vi "CalcStepUncertainty.vi"(8 "error in (no error)":errorcluster, 10 "Limits":dbl[][][](array[numeric])=[[[0.059450168900494, 0.0606065605190911, 0.056793034460449, 0.0377791964132806, 0.0387680244678906, 0.041509529284321, 0.0, 0.0], [0.0543254248656728, 0.0605582232708396, 0.0705532258276927, 0.0403341376210629, 0.0362750710120636, 0.037641124860868, 0.0, 0.0], [0.0542535208152999, 0.0601149006696316, 0.057100190511556, 0.0286705153398605, 0.0306659503421681, 0.0318434771124804, 0.0, 0.0], [0.0539806772823237, 0.060111916581221, 0.0568149701475802, 0.0287477348403936, 0.030687681069202, 0.0318140233011936, 0.0, 0.0], [0.0574739206185427, 0.0628177175852463, 0.0608742935192014, 0.0507031710323209, 0.0492196025001063, 0.0512494967622953, 0.0, 0.0], [0.0573743399751993, 0.0636926206100454, 0.0626583117825458, 0.0369031527657219, 0.0385466857090226, 0.0400368175447213, 0.0, 0.0], [0.0831820808794742, 0.0842623844587226, 0.088262229564689, 0.0667743079383481, 0.0680308099651913, 0.0679787518894359, 0.0, 0.0], [0.0541037185786453, 0.0597178605956032, 0.0641248041876747, 0.0281653525639868, 0.0301909812864416, 0.0304719216326717, 0.0, 0.0], [0.0564462783136314, 0.0600214622402702, 0.0759912985981658, 0.0281162118220652, 0.0301892901163339, 0.0303638978137465, 0.0, 0.0], [0.0540653703792215, 0.0598738420777627, 0.0612858805251609, 0.0282196395706911, 0.0301950277548319, 0.0310242020330342, 0.0, 0.0], [0.056709051486753, 0.0602058925674664, 0.0806981932623049, 0.0281451428430134, 0.0302542048015808, 0.0304691904137436, 0.0, 0.0]]], 11 "Uncertainties":dbl[][][](array[numeric])=[[[0.059450168900494, 0.0606065605190911, 0.056793034460449, 0.0377791964132806, 0.0387680244678906, 0.041509529284321, 0.0, 0.0], [0.0543254248656728, 0.0605582232708396, 0.0705532258276927, 0.0403341376210629, 0.0362750710120636, 0.037641124860868, 0.0, 0.0], [0.0542535208152999, 0.0601149006696316, 0.057100190511556, 0.0286705153398605, 0.0306659503421681, 0.0318434771124804, 0.0, 0.0], [0.0539806772823237, 0.060111916581221, 0.0568149701475802, 0.0287477348403936, 0.030687681069202, 0.0318140233011936, 0.0, 0.0], [0.0574739206185427, 0.0628177175852463, 0.0608742935192014, 0.0507031710323209, 0.0492196025001063, 0.0512494967622953, 0.0, 0.0], [0.0573743399751993, 0.0636926206100454, 0.0626583117825458, 0.0369031527657219, 0.0385466857090226, 0.0400368175447213, 0.0, 0.0], [0.0831820808794742, 0.0842623844587226, 0.088262229564689, 0.0667743079383481, 0.0680308099651913, 0.0679787518894359, 0.0, 0.0], [0.0541037185786453, 0.0597178605956032, 0.0641248041876747, 0.0281653525639868, 0.0301909812864416, 0.0304719216326717, 0.0, 0.0], [0.0564462783136314, 0.0600214622402702, 0.0759912985981658, 0.0281162118220652, 0.0301892901163339, 0.0303638978137465, 0.0, 0.0], [0.0540653703792215, 0.0598738420777627, 0.0612858805251609, 0.0282196395706911, 0.0301950277548319, 0.0310242020330342, 0.0, 0.0], [0.056709051486753, 0.0602058925674664, 0.0806981932623049, 0.0281451428430134, 0.0302542048015808, 0.0304691904137436, 0.0, 0.0]]]) -> (0 "error out":errorcluster, 1 "clDlyTime":T1, 2 "clOvrUndr":T2={"OvrUndr"=[[[[[5.598492295160192, 5.589160017980474, 5.579827740800756, 6.2090278478135055, 6.202935187769419, 6.196842527725332, 6.270368754436869, 6.261733208094874, 6.2530976617528795, 5.499241138114173, 5.4912209769255735, 5.483200815736974, 5.591363005137677, 5.589161707344972, 5.586960409552266, 6.2034021327898525, 6.2029551231392706, 6.202508113488689, 6.262186470202315, 6.261747037530138, 6.261307604857961, 5.492149609028501, 5.491120362323346, 5.490091115618191], [4.582281382800085, 4.572949105620367, 4.563616828440649, 2.0737377226338936, 2.0676450625898064, 2.0615524025457193, 1.1136472889469742, 1.1050117426049793, 1.0963761962629843, 4.500837324127726, 4.492817162939127, 4.484797001750527, 4.57515178562041, 4.572950487827704, 4.570749190034999, 2.068098717363672, 2.06765170771309, 2.067204698062508, 1.1054536157657309, 1.1050141830935536, 1.1045747504213763, 4.493764088606066, 4.492734841900911, 4.491705595195756], [6.26023399342542, 6.250901716245702, 6.241569439065984, 6.128438171518977, 6.12234551147489, 6.116252851430803, 6.430675694174775, 6.422040147832781, 6.413404601490786, 6.102855597590311, 6.094835436401712, 6.086815275213112, 6.253149166340811, 6.2509478685481055, 6.2487465707554, 6.122858708702316, 6.122411699051734, 6.121964689401152, 6.422526817417168, 6.422087384744991, 6.421647952072814, 6.095816462969536, 6.094787216264381, 6.093757969559226], [3.375202432081235, 3.3658701549015175, 3.3565378777218, 3.302740243145951, 3.296647583101864, 3.2905549230577766, 1.1419367489007164, 1.1333012025587215, 1.1246656562167265, 2.0396319733224955, 2.0316118121338955, 2.0235916509452956, 3.368096303933992, 3.3658950061412862, 3.3636937083485803, 3.297130232216894, 3.296683222566312, 3.29623621291573, 1.1337489711565862, 1.133309538484409, 1.1328701058122317, 2.0326249854599556, 2.0315957387548007, 2.030566492049646]], [[5.6114389386325305, 5.602495822485004, 5.593552706337477, 6.4971644746473425, 6.4906779148884395, 6.4841913551295365, 6.452789687138199, 6.442635198982573, 6.432480710826947, 5.499700075652654, 5.491172020965302, 5.4826439662779505, 5.604365790119637, 5.602470106718821, 5.600574423318005, 6.491501742716185, 6.490751963178685, 6.4900021836411845, 6.443115798655941, 6.442548550239463, 6.4419813018229855, 5.492187667629821, 5.4911167638448894, 5.490045860059958], [4.592803334544344, 4.583860218396818, 4.574917102249291, 1.1519003094451032, 1.1454137496861998, 1.1389271899272964, 2.1576995544831505, 2.147545066327524, 2.1373905781718974, 4.501305162749851, 4.4927771080625, 4.484249053375148, 4.585734861625306, 4.58383917822449, 4.5819434948236735, 1.146176596569033, 1.1454268170315325, 1.144677037494032, 2.148083431829625, 2.1475161834131473, 2.1469489349966695, 4.4938028014762015, 4.49273189769127, 4.491660993906338], [5.824200079831354, 5.815256963683828, 5.806313847536301, 6.213851725577966, 6.207365165819063, 6.20087860606016, 6.175131282852548, 6.164976794696922, 6.154822306541296, 6.103387438698514, 6.094859384011162, 6.08633132932381, 5.81714404673894, 5.815248363338124, 5.813352679937307, 6.208174990295637, 6.207425210758137, 6.206675431220637, 6.165428416601619, 6.1648611681851415, 6.164293919768664, 6.095893577165425, 6.094822673380493, 6.093751769595562], [3.140235327361881, 3.1312922112143546, 3.1223490950668285, 1.101903941962272, 1.0954173822033686, 1.0889308224444652, 2.0651467530546004, 2.054992264898974, 2.044837776743347, 2.040147849357748, 2.0316197946703958, 2.0230917399830437, 3.133183263659809, 3.131287580258993, 3.1293918968581766, 1.0961777579065755, 1.095427978369075, 1.0946781988315746, 2.0555209711448583, 2.0549537227283805, 2.0543864743119027, 2.032678461578429, 2.0316075577934978, 2.0305366540085665]]]]], "OvrUndrPFI"=[]} {"OvrUndr" format="%_3g"}, 3 "Step Error":dbl[][][][][](array[numeric]), 5 "clRespTime":T3 {"RT Uncert" format="%#_2g"; "RT Range" format="%#_4g"}, 7 "StepData":dbl[][][][][](array[numeric]))   [LabVIEW 2014]
uses:
  typedef/PMUConfig.ctl
panel:
  # "VA"
  # "VB"
  # "VC"
  # "V+"
  # "IA"
  # "IB"
  # "IC"
  # "I+"
  # "Phase Step Pos"
  # "Phase Step Neg"
  # "Mag Step Pos"
  # "Mag Step Neg"
  # "VA"
  # "VB"
  # "VC"
  # "V+"
  # "IA"
  # "IB"
  # "IC"
  # "I+"
  # "DT + Unc"
  # "DT"
  # "DT - Unc"
  # "VA"
  # "VB"
  # "VC"
  # "V+"
  # "IA"
  # "IB"
  # "IC"
  # "I+"
  # "PreOvr"
  # "PreUndr"
  # "PostOvr"
  # "PostUndr"
  # "VA+u"
  # "VA"
  # "VA-u"
  # "VBu"
  # "VB"
  # "VB-u"
  # "VCu"
  # "VCB"
  # "VC-u"
  # "V+u"
  # "V+B"
  # "V+-u"
  # "IA+u"
  # "IA"
  # "IA-u"
  # "IBu"
  # "IB"
  # "IB-u"
  # "ICu"
  # "ICB"
  # "IC-u"
  # "I+u"
  # "I+B"
  # "I+-u"
  # "PreOvr"
  # "PreUndr"
  # "PostOvr"
  # "PostUndr"
  # "VB"
  # "FREQ"
  # "VA"
  # "VC"
  # "V+"
  # "IA"
  # "IB"
  # "IC"
  # "I+"
  # "ROCOF"
  # "Phase Step Positive"
  # "Phase Step Negative"
  # "Mag Step Positive"
  # "Mag Step Negative"
  # "plus\n\nRT\n\nminus"
  # "RT + unc\n\nRT\n\nRT - unc"
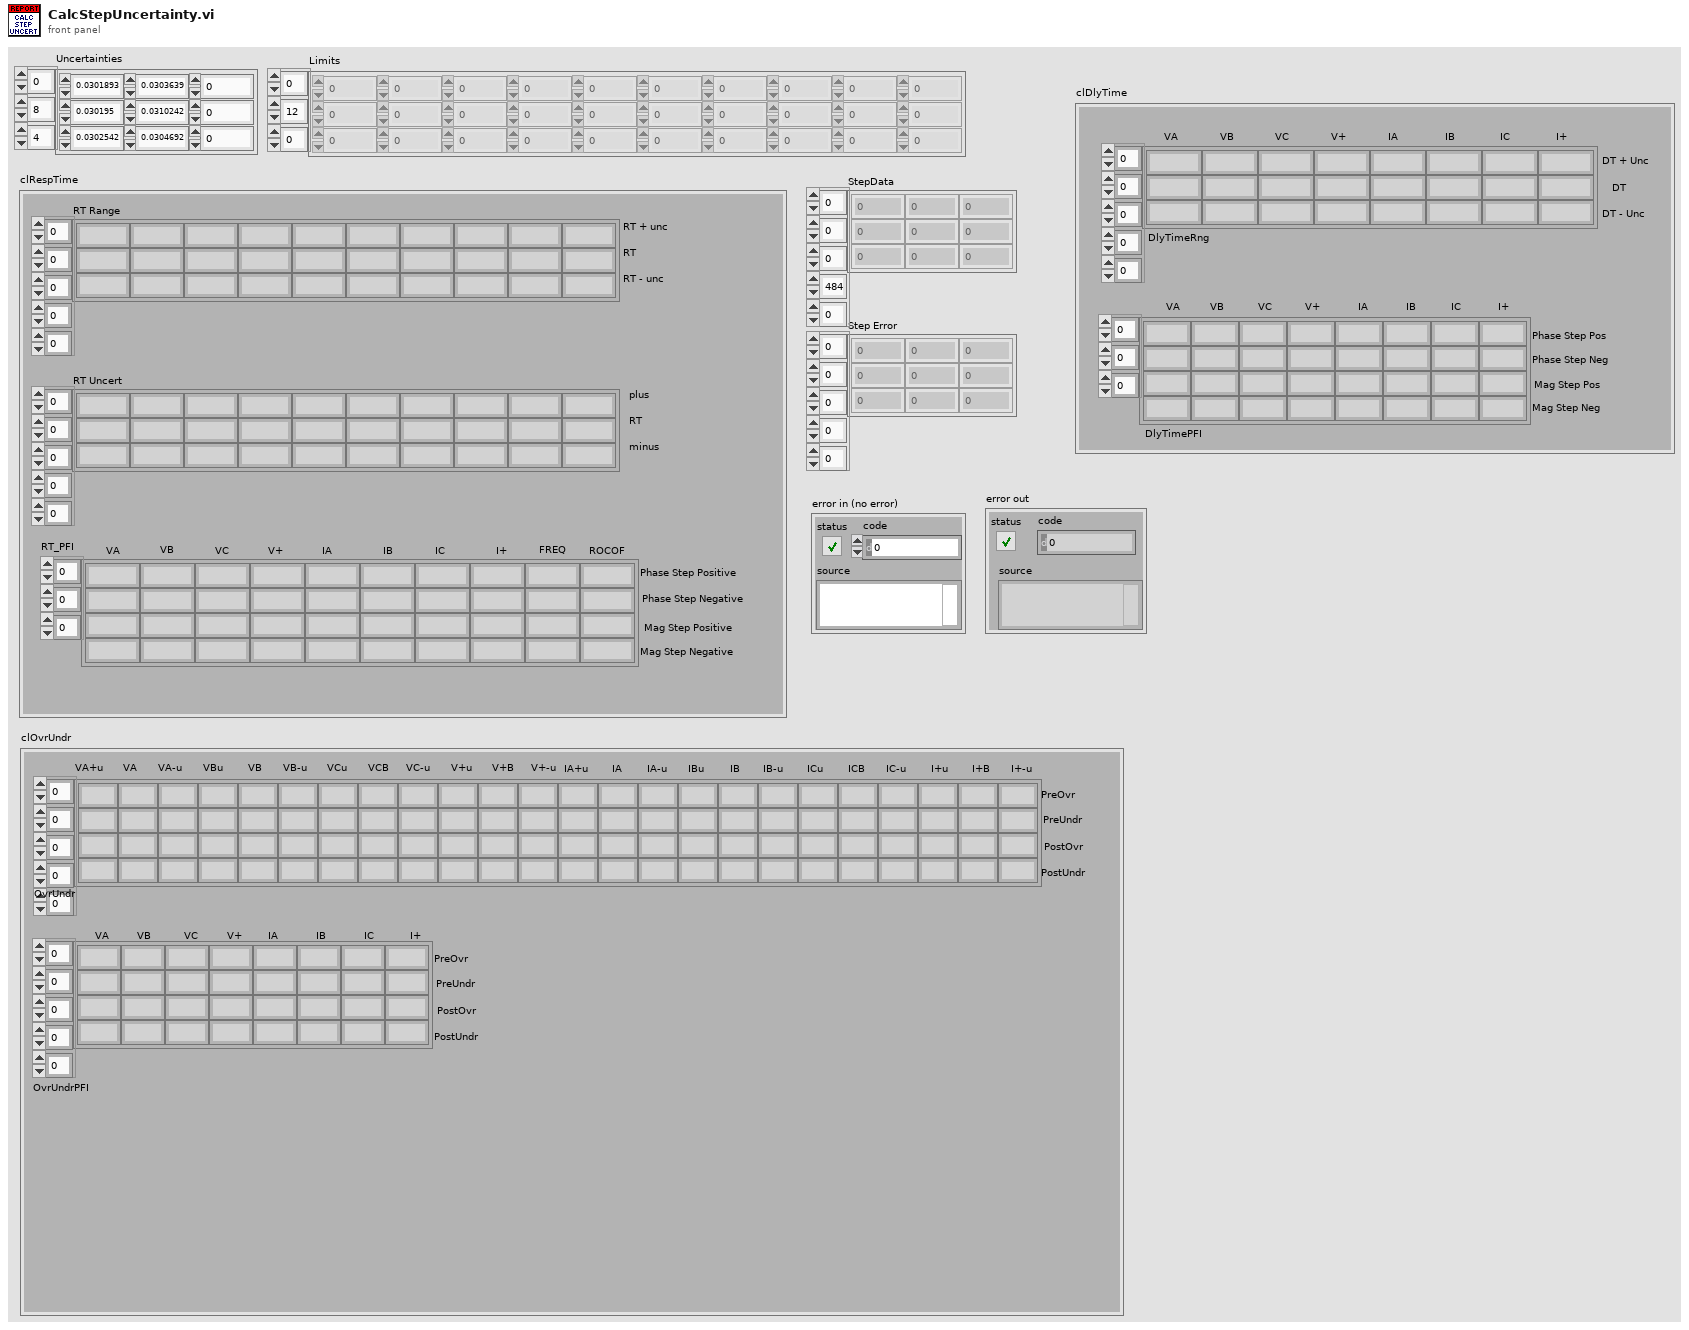
[diagram p1: front panel]
types:
  T1 = cluster{"DlyTimeRng":dbl[][][][][], "DlyTimePFI":string[][][]}
  T2 = cluster{"OvrUndr":dbl[][][][][], "OvrUndrPFI":string[][][][][]}
  T3 = cluster{"RT Range":dbl[][][][][], "RT Uncert":dbl[][][][][], "RT_PFI":string[][][]}
  T4 = typedef "PMUConfig.ctl" = cluster{"Class":string, "Fs":dbl, "F0":dbl}
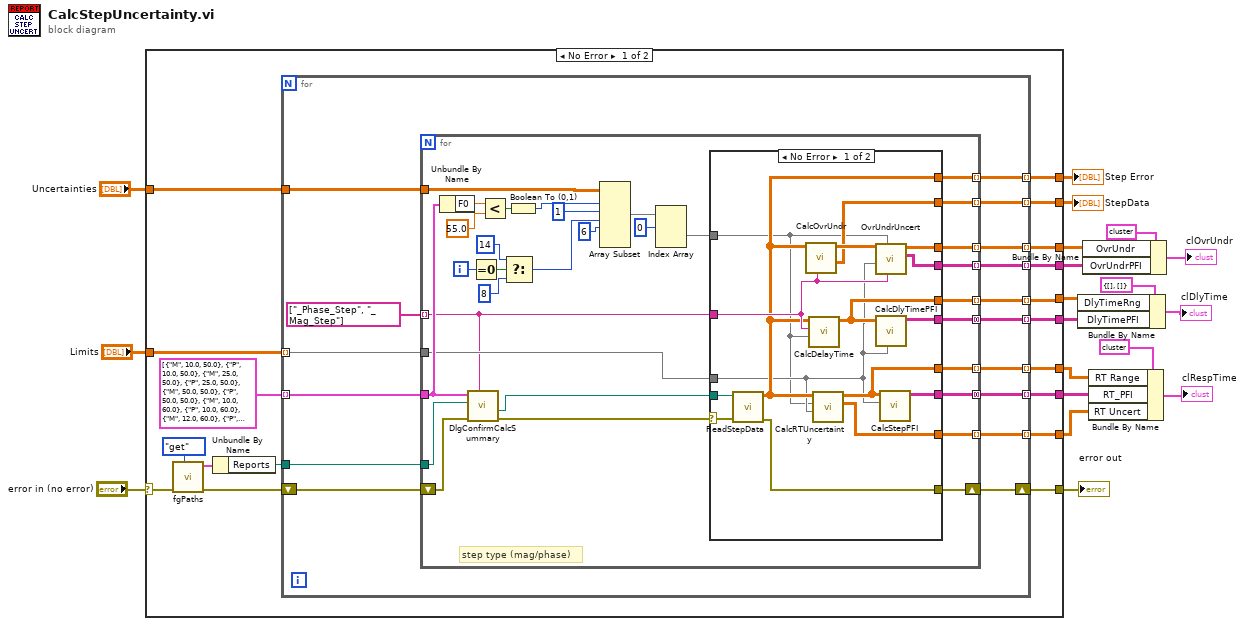
[diagram p0: block diagram]
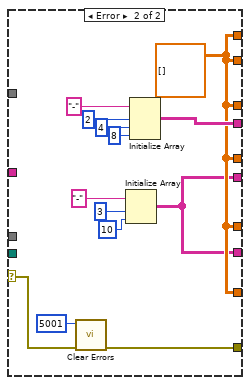
[diagram p2: hidden frame]
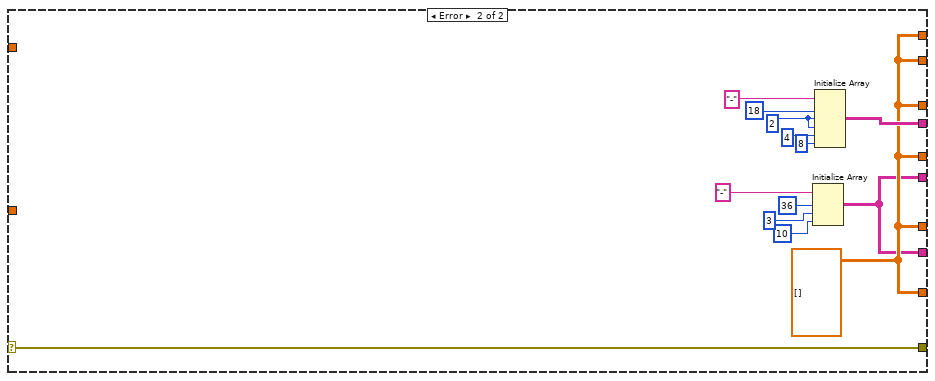
[diagram p3: hidden frame]
diagram:
  n1 = case shown="No Error" "error in (no error)" {
    selector: "error in (no error)" -> [w34 w127]
    tunnel: [w32 w127] -> w18
    tunnel: [w30 w115] -> w10
    tunnel: [w29 w116] -> w13
    tunnel: [w28 w116] -> w9
    tunnel: "Uncertainties" -> [w27 _]
    tunnel: "Limits" -> [w26 _]
    tunnel: [w25 w116] -> w15
    tunnel: [w24 w116] -> w6
    tunnel: [w23 w121] -> w5
    tunnel: [w22 w116] -> w14
    tunnel: [w21 w115] -> w2
    tunnel: [w20 w116] -> w3
    frame No Error {
      n2 = call "fgPaths.vi"("cmd"=enum16{"init", "set", "get"}."get", "error in (no error)"=w34) -> ("error out"=w33:errorcluster, "clPaths"=w35:cluster{"Templates":path, "Reports":path})  [unwired: 8 in]
      n3 = Unbundle By Name(w35) -> ("Reports"=w31:path)
      n4 = for {
        tunnel: T4[] [{"Class"="M", "Fs"=10.0, "F0"=50.0}, {"Class"="P", "Fs"=10.0, "F0"=50.0}, {"Class"="M", "Fs"=25.0, "F0"=50.0}, {"Class"="P", "Fs"=25.0, "F0"=50.0}, {"Class"="M", "Fs"=50.0, "F0"=50.0}, {"Class"="P", "Fs"=50.0, "F0"=50.0}, {"Class"="M", "Fs"=10.0, "F0"=60.0}, {"Class"="P", "Fs"=10.0, "F0"=60.0}, {"Class"="M", "Fs"=12.0, "F0"=60.0}, {"Class"="P", "Fs"=12.0, "F0"=60.0}, {"Class"="M", "Fs"=15.0, "F0"=60.0}, {"Class"="P", "Fs"=15.0, "F0"=60.0}, {"Class"="M", "Fs"=20.0, "F0"=60.0}, {"Class"="P", "Fs"=20.0, "F0"=60.0}, {"Class"="M", "Fs"=30.0, "F0"=60.0}, {"Class"="P", "Fs"=30.0, "F0"=60.0}, {"Class"="M", "Fs"=60.0, "F0"=60.0}, {"Class"="P", "Fs"=60.0, "F0"=60.0}] -> [w52] mode=indexing
        shift-right: [w50] -> w32
        shift-left: w33 -> [w51]
        tunnel: w31 -> [w49]
        tunnel: [w48] -> w30 mode=indexing
        tunnel: [w47] -> w29 mode=indexing
        tunnel: [w46] -> w28 mode=indexing
        tunnel: w27 -> [w45]
        tunnel: w26 -> [w44] mode=indexing
        tunnel: [w43] -> w25 mode=indexing
        tunnel: [w42] -> w24 mode=indexing
        tunnel: [w41] -> w23 mode=indexing
        tunnel: [w40] -> w22 mode=indexing
        tunnel: [w39] -> w21 mode=indexing
        tunnel: [w38] -> w20 mode=indexing
        n5 = for {
          tunnel: string[] ["_Phase_Step", "_Mag_Step"] -> [w59] mode=indexing
          tunnel: w52 -> [w74]
          shift-right: [w81] -> w50
          shift-left: w51 -> [w85]
          tunnel: w49 -> [w84]
          tunnel: [w82] -> w48 mode=concatenating
          tunnel: [w80] -> w47 mode=indexing
          tunnel: [w79] -> w46 mode=indexing
          tunnel: w45 -> [w70]
          tunnel: w44 -> [w60]
          tunnel: [w61] -> w43 mode=indexing
          tunnel: [w58] -> w42 mode=indexing
          tunnel: [w57] -> w41 mode=indexing
          tunnel: [w56] -> w40 mode=indexing
          tunnel: [w55] -> w39 mode=concatenating
          tunnel: [w54] -> w38 mode=indexing
          i -> [w78]
          # "step type (mag/phase)"
          n6 = Unbundle By Name(w74) -> ("F0"=w73:dbl)
          n7 = call "DlgConfirmCalcSummary.vi"("Suffix"=w59, "error in (no error)"=w85, "Path"=w84, "PMUConfig"=w74) -> ("error out"=w83:errorcluster, "Summary Data Excel File"=w63:path)  [unwired: 4 in, 2 out]
          n8 = Equal To 0?(x=w78) -> (x = 0?=w77:bool)
          n9 = Less?(x=w73, y=55.0) -> (x < y?=w71:bool)
          n10 = Select(t=14, s=w77, f=8) -> (s? t:f=w64:i32)
          n11 = Boolean To (0,1)(Boolean=w71) -> (0, 1=w69:i16)
          n12 = Array Subset(array=w70, index (dim 0)=w69, length (dim 0)=1 ("length"), index (dim 1)=w64, length (dim 1)=6 ("length")) -> (w67:dbl[][][])  [unwired: 2 in]
          n13 = Index Array(array=w67, index (dim 0)=0 ("index (page)")) -> (element=w65:dbl[][])  [unwired: 2 in]
          n14 = case shown="No Error" w83 {
            selector: w83 -> [w101 w113]
            tunnel: [w96 w102] -> w82
            tunnel: [w98 w109] -> w81
            tunnel: [w97 w103] -> w80
            tunnel: [w99 w103] -> w79
            tunnel: w65 -> [w86 _]
            tunnel: w63 -> [w100 _]
            tunnel: [w90 w103] -> w61
            tunnel: w60 -> [w87 _]
            tunnel: w59 -> [w91 _]
            tunnel: [w94 w103] -> w58
            tunnel: [w93 w108] -> w57
            tunnel: [w92 w103] -> w56
            tunnel: [w89 w102] -> w55
            tunnel: [w88 w103] -> w54
            frame No Error {
              n15 = call "ReadStepData.vi"("error in (no error)"=w101, "DataPath"=w100) -> ("error out"=w98:errorcluster, "Step Data"=w90:dbl[][][])  [unwired: 6 in, 1 out]
              n16 = call "CalcOvrUndr.vi"("StepType"=w91, "Step Data"=w90) -> ("StepData"=w92:dbl[][][], "OvrUndr"=w95:dbl[][][])  [unwired: 7 in, 1 out]
              n17 = call "CalcDelayTime.vi"("Uncertainties"=w86, "StepType"=w91, "Step Data"=w90) -> ("DelayTime Range"=w88:dbl[][][])  [unwired: 8 in]
              n18 = call "CalcRTUncertainty.vi"("Limits"=w87, "Uncertainties"=w86, "Step Data"=w90) -> ("Uncert"=w99:dbl[][][], "Range"=w97:dbl[][][])  [unwired: 7 in]
              n19 = call "OvrUndrUncert.vi"("StepType"=w91, "Uncert"=w86, "Limits"=w87, "OvrUndr"=w95) -> ("PFI"=w93:string[][][], "OvrUndr"=w94:dbl[][][])  [unwired: 6 in]
              n20 = call "CalcDlyTimePFI.vi"("Limits"=w87, "Results"=w88) -> ("PFI"=w89:string[][])  [unwired: 9 in]
              n21 = call "CalcStepPFI.vi"("Limits"=w87, "Results"=w97) -> ("PFI"=w96:string[][])  [unwired: 9 in]
            }
            frame Error {
              w103 = dbl[][][] [] ("Step Data")
              n22 = call <vilib>:"Clear Errors.vi"("error in (no error)"=w113, "specific error code to clear (0: all)"=5001) -> ("error out"=w109:errorcluster)  [unwired: 4 in, 1 out]
              n23 = Initialize Array("-", 3 ("dimension size"), 10 ("dimension size")) -> (w102:string[][])
              n24 = Initialize Array("-", 2 ("dimension size"), 4 ("dimension size"), 8 ("dimension size")) -> (w108:string[][][])
            }
          }
        }
      }
    }
    frame Error {
      w117 = 2 ("dimension size")
      w116 = dbl[][][][][] [] ("Results")
      n25 = Initialize Array("-", 36 ("dimension size"), 3 ("dimension size"), 10 ("dimension size")) -> (w115:string[][][])
      n26 = Initialize Array("-", 18 ("dimension size"), w117, w117, 4 ("dimension size"), 8 ("dimension size")) -> (w121:string[][][][][])
    }
  }
  "error out" <- w18
  "Step Error" <- w15
  "StepData" <- w14
  n27 = Bundle By Name(cluster=T1 {"DlyTimeRng"=[], "DlyTimePFI"=[]} ("input cluster"), "DlyTimeRng"=w3, "DlyTimePFI"=w2) -> (→"clDlyTime":T1)
  n28 = Bundle By Name(cluster=T2 {"OvrUndr"=array18x2x2x4x24[6912 elements], "OvrUndrPFI"=[[[[["P", "P", "P", "P", "P", "P", "P", "P"], ["P", "P", "P", "P", "P", "P", "P", "P"], ["P", "P", "P", "P", "P", "P", "P", "P"], ["P", "P", "P", "P", "P", "P", "P", "P"]], [["P", "P", "P", "P", "P", "P", "P", "P"], ["P", "P", "P", "P", "P", "P", "P", "P"], ["P", "P", "P", "P", "P", "P", "P", "P"], ["P", "P", "P", "P", "P", "P", "P", "P"]]], [[["P", "P", "P", "P", "P", "P", "P", "P"], ["P", "P", "P", "P", "P", "P", "P", "P"], ["P", "P", "P", "P", "P", "P", "P", "P"], ["P", "P", "P", "P", "P", "P", "P", "P"]], [["P", "P", "P", "P", "P", "P", "P", "P"], ["P", "P", "P", "P", "P", "P", "P", "P"], ["P", "P", "P", "P", "P", "P", "P", "P"], ["P", "P", "P", "P", "P", "P", "P", "P"]]]], [[[["P", "P", "P", "P", "P", "P", "P", "P"], ["P", "P", "P", "P", "P", "P", "P", "P"], ["P", "P", "P", "P", "P", "P", "P", "P"], ["P", "P", "P", "P", "P", "P", "P", "P"]], [["P", "P", "P", "P", "P", "P", "P", "P"], ["P", "P", "P", "P", "P", "P", "P", "P"], ["P", "P", "P", "P", "P", "P", "P", "P"], ["P", "P", "P", "P", "P", "P", "P", "P"]]], [[["P", "P", "P", "P", "P", "P", "P", "P"], ["P", "P", "P", "P", "P", "P", "P", "P"], ["P", "P", "P", "P", "P", "P", "P", "P"], ["P", "P", "P", "P", "P", "P", "P", "P"]], [["P", "P", "P", "P", "P", "P", "P", "P"], ["P", "P", "P", "P", "P", "P", "P", "P"], ["P", "P", "P", "P", "P", "P", "P", "P"], ["P", "P", "P", "P", "P", "P", "P", "P"]]]], [[[["P", "P", "P", "P", "P", "P", "P", "P"], ["P", "P", "P", "P", "P", "P", "P", "P"], ["P", "P", "P", "P", "P", "P", "P", "P"], ["P", "P", "P", "P", "P", "P", "P", "P"]], [["P", "P", "P", "P", "P", "P", "P", "P"], ["P", "P", "P", "P", "P", "P", "P", "P"], ["P", "P", "P", "P", "P", "P", "P", "P"], ["P", "P", "P", "P", "P", "P", "P", "P"]]], [[["P", "P", "P", "P", "P", "P", "P", "P"], ["P", "P", "P", "P", "P", "P", "P", "P"], ["P", "P", "P", "P", "P", "P", "P", "P"], ["P", "P", "P", "P", "P", "P", "P", "P"]], [["P", "P", "P", "P", "P", "P", "P", "P"], ["P", "P", "P", "P", "P", "P", "P", "P"], ["P", "P", "P", "P", "P", "P", "P", "P"], ["P", "P", "P", "P", "P", "P", "P", "P"]]]], [[[["P", "P", "P", "P", "P", "P", "P", "P"], ["P", "P", "P", "P", "P", "P", "P", "P"], ["P", "P", "P", "P", "P", "P", "P", "P"], ["P", "P", "P", "P", "P", "P", "P", "P"]], [["P", "P", "P", "P", "P", "P", "P", "P"], ["P", "P", "P", "P", "P", "P", "P", "P"], ["P", "P", "P", "P", "P", "P", "P", "P"], ["P", "P", "P", "P", "P", "P", "P", "P"]]], [[["P", "P", "P", "P", "P", "P", "P", "P"], ["P", "P", "P", "P", "P", "P", "P", "P"], ["P", "P", "P", "P", "P", "P", "P", "P"], ["P", "P", "P", "P", "P", "P", "P", "P"]], [["P", "P", "P", "P", "P", "P", "P", "P"], ["P", "P", "P", "P", "P", "P", "P", "P"], ["P", "P", "P", "P", "P", "P", "P", "P"], ["P", "P", "P", "P", "P", "P", "P", "P"]]]], [[[["P", "P", "P", "P", "P", "P", "P", "P"], ["P", "P", "P", "P", "P", "P", "P", "P"], ["P", "P", "P", "P", "P", "P", "P", "P"], ["P", "P", "P", "P", "P", "P", "P", "P"]], [["P", "P", "P", "P", "P", "P", "P", "P"], ["P", "P", "P", "P", "P", "P", "P", "P"], ["P", "P", "P", "P", "P", "P", "P", "P"], ["P", "P", "P", "P", "P", "P", "P", "P"]]], [[["P", "P", "P", "P", "P", "P", "P", "P"], ["P", "P", "P", "P", "P", "P", "P", "P"], ["P", "P", "P", "P", "P", "P", "P", "P"], ["P", "P", "P", "P", "P", "P", "P", "P"]], [["P", "P", "P", "P", "P", "P", "P", "P"], ["P", "P", "P", "P", "P", "P", "P", "P"], ["P", "P", "P", "P", "P", "P", "P", "P"], ["P", "P", "P", "P", "P", "P", "P", "P"]]]], [[[["P", "P", "P", "P", "P", "P", "P", "P"], ["P", "P", "P", "P", "P", "P", "P", "P"], ["P", "P", "P", "P", "P", "P", "P", "P"], ["P", "P", "P", "P", "P", "P", "P", "P"]], [["P", "P", "P", "P", "P", "P", "P", "P"], ["P", "P", "P", "P", "P", "P", "P", "P"], ["P", "P", "P", "P", "P", "P", "P", "P"], ["P", "P", "P", "P", "P", "P", "P", "P"]]], [[["P", "P", "P", "P", "P", "P", "P", "P"], ["P", "P", "P", "P", "P", "P", "P", "P"], ["P", "P", "P", "P", "P", "P", "P", "P"], ["P", "P", "P", "P", "P", "P", "P", "P"]], [["P", "P", "P", "P", "P", "P", "P", "P"], ["P", "P", "P", "P", "P", "P", "P", "P"], ["P", "P", "P", "P", "P", "P", "P", "P"], ["P", "P", "P", "P", "P", "P", "P", "P"]]]], [[[["P", "P", "P", "P", "P", "P", "P", "P"], ["P", "P", "P", "P", "P", "P", "P", "P"], ["P", "P", "P", "P", "P", "P", "P", "P"], ["P", "P", "P", "P", "P", "P", "P", "P"]], [["P", "P", "P", "P", "P", "P", "P", "P"], ["P", "P", "P", "P", "P", "P", "P", "P"], ["P", "P", "P", "P", "P", "P", "P", "P"], ["P", "P", "P", "P", "P", "P", "P", "P"]]], [[["P", "P", "P", "P", "P", "P", "P", "P"], ["P", "P", "P", "P", "P", "P", "P", "P"], ["P", "P", "P", "P", "P", "P", "P", "P"], ["P", "P", "P", "P", "P", "P", "P", "P"]], [["P", "P", "P", "P", "P", "P", "P", "P"], ["P", "P", "P", "P", "P", "P", "P", "P"], ["P", "P", "P", "P", "P", "P", "P", "P"], ["P", "P", "P", "P", "P", "P", "P", "P"]]]], [[[["P", "P", "P", "P", "P", "P", "P", "P"], ["P", "P", "P", "P", "P", "P", "P", "P"], ["P", "P", "P", "P", "P", "P", "P", "P"], ["P", "P", "P", "P", "P", "P", "P", "P"]], [["P", "P", "P", "P", "P", "P", "P", "P"], ["P", "P", "P", "P", "P", "P", "P", "P"], ["P", "P", "P", "P", "P", "P", "P", "P"], ["P", "P", "P", "P", "P", "P", "P", "P"]]], [[["P", "P", "P", "P", "P", "P", "P", "P"], ["P", "P", "P", "P", "P", "P", "P", "P"], ["P", "P", "P", "P", "P", "P", "P", "P"], ["P", "P", "P", "P", "P", "P", "P", "P"]], [["P", "P", "P", "P", "P", "P", "P", "P"], ["P", "P", "P", "P", "P", "P", "P", "P"], ["P", "P", "P", "P", "P", "P", "P", "P"], ["P", "P", "P", "P", "P", "P", "P", "P"]]]], [[[["P", "P", "P", "P", "P", "P", "P", "P"], ["P", "P", "P", "P", "P", "P", "P", "P"], ["P", "P", "P", "P", "P", "P", "P", "P"], ["P", "P", "P", "P", "P", "P", "P", "P"]], [["P", "P", "P", "P", "P", "P", "P", "P"], ["P", "P", "P", "P", "P", "P", "P", "P"], ["P", "P", "P", "P", "P", "P", "P", "P"], ["P", "P", "P", "P", "P", "P", "P", "P"]]], [[["P", "P", "P", "P", "P", "P", "P", "P"], ["P", "P", "P", "P", "P", "P", "P", "P"], ["P", "P", "P", "P", "P", "P", "P", "P"], ["P", "P", "P", "P", "P", "P", "P", "P"]], [["P", "P", "P", "P", "P", "P", "P", "P"], ["P", "P", "P", "P", "P", "P", "P", "P"], ["P", "P", "P", "P", "P", "P", "P", "P"], ["P", "P", "P", "P", "P", "P", "P", "P"]]]], [[[["P", "P", "P", "P", "P", "P", "P", "P"], ["P", "P", "P", "P", "P", "P", "P", "P"], ["P", "P", "P", "P", "P", "P", "P", "P"], ["P", "P", "P", "P", "P", "P", "P", "P"]], [["P", "P", "P", "P", "P", "P", "P", "P"], ["P", "P", "P", "P", "P", "P", "P", "P"], ["P", "P", "P", "P", "P", "P", "P", "P"], ["P", "P", "P", "P", "P", "P", "P", "P"]]], [[["P", "P", "P", "P", "P", "P", "P", "P"], ["P", "P", "P", "P", "P", "P", "P", "P"], ["P", "P", "P", "P", "P", "P", "P", "P"], ["P", "P", "P", "P", "P", "P", "P", "P"]], [["P", "P", "P", "P", "P", "P", "P", "P"], ["P", "P", "P", "P", "P", "P", "P", "P"], ["P", "P", "P", "P", "P", "P", "P", "P"], ["P", "P", "P", "P", "P", "P", "P", "P"]]]], [[[["P", "P", "P", "P", "P", "P", "P", "P"], ["P", "P", "P", "P", "P", "P", "P", "P"], ["P", "P", "P", "P", "P", "P", "P", "P"], ["P", "P", "P", "P", "P", "P", "P", "P"]], [["P", "P", "P", "P", "P", "P", "P", "P"], ["P", "P", "P", "P", "P", "P", "P", "P"], ["P", "P", "P", "P", "P", "P", "P", "P"], ["P", "P", "P", "P", "P", "P", "P", "P"]]], [[["P", "P", "P", "P", "P", "P", "P", "P"], ["P", "P", "P", "P", "P", "P", "P", "P"], ["P", "P", "P", "P", "P", "P", "P", "P"], ["P", "P", "P", "P", "P", "P", "P", "P"]], [["P", "P", "P", "P", "P", "P", "P", "P"], ["P", "P", "P", "P", "P", "P", "P", "P"], ["P", "P", "P", "P", "P", "P", "P", "P"], ["P", "P", "P", "P", "P", "P", "P", "P"]]]], [[[["P", "P", "P", "P", "P", "P", "P", "P"], ["P", "P", "P", "P", "P", "P", "P", "P"], ["P", "P", "P", "P", "P", "P", "P", "P"], ["P", "P", "P", "P", "P", "P", "P", "P"]], [["P", "P", "P", "P", "P", "P", "P", "P"], ["P", "P", "P", "P", "P", "P", "P", "P"], ["P", "P", "P", "P", "P", "P", "P", "P"], ["P", "P", "P", "P", "P", "P", "P", "P"]]], [[["P", "P", "P", "P", "P", "P", "P", "P"], ["P", "P", "P", "P", "P", "P", "P", "P"], ["P", "P", "P", "P", "P", "P", "P", "P"], ["P", "P", "P", "P", "P", "P", "P", "P"]], [["P", "P", "P", "P", "P", "P", "P", "P"], ["P", "P", "P", "P", "P", "P", "P", "P"], ["P", "P", "P", "P", "P", "P", "P", "P"], ["P", "P", "P", "P", "P", "P", "P", "P"]]]], [[[["P", "P", "P", "P", "P", "P", "P", "P"], ["P", "P", "P", "P", "P", "P", "P", "P"], ["P", "P", "P", "P", "P", "P", "P", "P"], ["P", "P", "P", "P", "P", "P", "P", "P"]], [["P", "P", "P", "P", "P", "P", "P", "P"], ["P", "P", "P", "P", "P", "P", "P", "P"], ["P", "P", "P", "P", "P", "P", "P", "P"], ["P", "P", "P", "P", "P", "P", "P", "P"]]], [[["P", "P", "P", "P", "P", "P", "P", "P"], ["P", "P", "P", "P", "P", "P", "P", "P"], ["P", "P", "P", "P", "P", "P", "P", "P"], ["P", "P", "P", "P", "P", "P", "P", "P"]], [["P", "P", "P", "P", "P", "P", "P", "P"], ["P", "P", "P", "P", "P", "P", "P", "P"], ["P", "P", "P", "P", "P", "P", "P", "P"], ["P", "P", "P", "P", "P", "P", "P", "P"]]]], [[[["P", "P", "P", "P", "P", "P", "P", "P"], ["P", "P", "P", "P", "P", "P", "P", "P"], ["P", "P", "P", "P", "P", "P", "P", "P"], ["P", "P", "P", "P", "P", "P", "P", "P"]], [["P", "P", "P", "P", "P", "P", "P", "P"], ["P", "P", "P", "P", "P", "P", "P", "P"], ["P", "P", "P", "P", "P", "P", "P", "P"], ["P", "P", "P", "P", "P", "P", "P", "P"]]], [[["P", "P", "P", "P", "P", "P", "P", "P"], ["P", "P", "P", "P", "P", "P", "P", "P"], ["P", "P", "P", "P", "P", "P", "P", "P"], ["P", "P", "P", "P", "P", "P", "P", "P"]], [["P", "P", "P", "P", "P", "P", "P", "P"], ["P", "P", "P", "P", "P", "P", "P", "P"], ["P", "P", "P", "P", "P", "P", "P", "P"], ["P", "P", "P", "P", "P", "P", "P", "P"]]]], [[[["P", "P", "P", "P", "P", "P", "P", "P"], ["P", "P", "P", "P", "P", "P", "P", "P"], ["P", "P", "P", "P", "P", "P", "P", "P"], ["P", "P", "P", "P", "P", "P", "P", "P"]], [["P", "P", "P", "P", "P", "P", "P", "P"], ["P", "P", "P", "P", "P", "P", "P", "P"], ["P", "P", "P", "P", "P", "P", "P", "P"], ["P", "P", "P", "P", "P", "P", "P", "P"]]], [[["P", "P", "P", "P", "P", "P", "P", "P"], ["P", "P", "P", "P", "P", "P", "P", "P"], ["P", "P", "P", "P", "P", "P", "P", "P"], ["P", "P", "P", "P", "P", "P", "P", "P"]], [["P", "P", "P", "P", "P", "P", "P", "P"], ["P", "P", "P", "P", "P", "P", "P", "P"], ["P", "P", "P", "P", "P", "P", "P", "P"], ["P", "P", "P", "P", "P", "P", "P", "P"]]]], [[[["P", "P", "P", "P", "P", "P", "P", "P"], ["P", "P", "P", "P", "P", "P", "P", "P"], ["P", "P", "P", "P", "P", "P", "P", "P"], ["P", "P", "P", "P", "P", "P", "P", "P"]], [["P", "P", "P", "P", "P", "P", "P", "P"], ["P", "P", "P", "P", "P", "P", "P", "P"], ["P", "P", "P", "P", "P", "P", "P", "P"], ["P", "P", "P", "P", "P", "P", "P", "P"]]], [[["P", "P", "P", "P", "P", "P", "P", "P"], ["P", "P", "P", "P", "P", "P", "P", "P"], ["P", "P", "P", "P", "P", "P", "P", "P"], ["P", "P", "P", "P", "P", "P", "P", "P"]], [["P", "P", "P", "P", "P", "P", "P", "P"], ["P", "P", "P", "P", "P", "P", "P", "P"], ["P", "P", "P", "P", "P", "P", "P", "P"], ["P", "P", "P", "P", "P", "P", "P", "P"]]]], [[[["P", "P", "P", "P", "P", "P", "P", "P"], ["P", "P", "P", "P", "P", "P", "P", "P"], ["P", "P", "P", "P", "P", "P", "P", "P"], ["P", "P", "P", "P", "P", "P", "P", "P"]], [["P", "P", "P", "P", "P", "P", "P", "P"], ["P", "P", "P", "P", "P", "P", "P", "P"], ["P", "P", "P", "P", "P", "P", "P", "P"], ["P", "P", "P", "P", "P", "P", "P", "P"]]], [[["P", "P", "P", "P", "P", "P", "P", "P"], ["P", "P", "P", "P", "P", "P", "P", "P"], ["P", "P", "P", "P", "P", "P", "P", "P"], ["P", "P", "P", "P", "P", "P", "P", "P"]], [["P", "P", "P", "P", "P", "P", "P", "P"], ["P", "P", "P", "P", "P", "P", "P", "P"], ["P", "P", "P", "P", "P", "P", "P", "P"], ["P", "P", "P", "P", "P", "P", "P", "P"]]]], [[[["P", "P", "P", "P", "P", "P", "P", "P"], ["P", "P", "P", "P", "P", "P", "P", "P"], ["P", "P", "P", "P", "P", "P", "P", "P"], ["P", "P", "P", "P", "P", "P", "P", "P"]], [["P", "P", "P", "P", "P", "P", "P", "P"], ["P", "P", "P", "P", "P", "P", "P", "P"], ["P", "P", "P", "P", "P", "P", "P", "P"], ["P", "P", "P", "P", "P", "P", "P", "P"]]], [[["P", "P", "P", "P", "P", "P", "P", "P"], ["P", "P", "P", "P", "P", "P", "P", "P"], ["P", "P", "P", "P", "P", "P", "P", "P"], ["P", "P", "P", "P", "P", "P", "P", "P"]], [["P", "P", "P", "P", "P", "P", "P", "P"], ["P", "P", "P", "P", "P", "P", "P", "P"], ["P", "P", "P", "P", "P", "P", "P", "P"], ["P", "P", "P", "P", "P", "P", "P", "P"]]]]]} ("clOvrUndr"), "OvrUndr"=w6, "OvrUndrPFI"=w5) -> (→"clOvrUndr":T2)
  n29 = Bundle By Name(cluster=T3 {"RT Range"=array18x2x2x3x10[2160 elements], "RT Uncert"=array18x2x2x3x10[2160 elements], "RT_PFI"=[[["P", "P", "P", "P", "P", "P", "P", "P", "P", "P"], ["P", "P", "P", "P", "P", "P", "P", "P", "P", "P"], ["P", "P", "P", "P", "P", "P", "P", "P", "P", "P"], ["P", "P", "P", "P", "P", "P", "P", "P", "P", "P"]], [["P", "P", "P", "P", "P", "P", "P", "P", "P", "P"], ["P", "P", "P", "P", "P", "P", "P", "P", "P", "P"], ["P", "P", "P", "P", "P", "P", "P", "P", "P", "P"], ["P", "P", "P", "P", "P", "P", "P", "P", "P", "P"]], [["P", "P", "P", "P", "P", "P", "P", "P", "P", "P"], ["P", "P", "P", "P", "P", "P", "P", "P", "P", "P"], ["P", "P", "P", "P", "P", "P", "P", "P", "P", "P"], ["P", "P", "P", "P", "P", "P", "P", "P", "P", "P"]], [["P", "P", "P", "P", "P", "P", "P", "P", "P", "P"], ["P", "P", "P", "P", "P", "P", "P", "P", "P", "P"], ["P", "P", "P", "P", "P", "P", "P", "P", "P", "P"], ["P", "P", "P", "P", "P", "P", "P", "P", "P", "P"]], [["P", "P", "P", "P", "P", "P", "P", "P", "P", "P"], ["P", "P", "P", "P", "P", "P", "P", "P", "P", "P"], ["P", "P", "P", "P", "P", "P", "P", "P", "P", "P"], ["P", "P", "P", "P", "P", "P", "P", "P", "P", "P"]], [["P", "P", "P", "P", "P", "P", "P", "P", "P", "P"], ["P", "P", "P", "P", "P", "P", "P", "P", "P", "P"], ["P", "P", "P", "P", "P", "P", "P", "P", "P", "P"], ["P", "P", "P", "P", "P", "P", "P", "P", "P", "P"]], [["P", "P", "P", "P", "P", "P", "P", "P", "P", "P"], ["P", "P", "P", "P", "P", "P", "P", "P", "P", "P"], ["P", "P", "P", "P", "P", "P", "P", "P", "P", "P"], ["P", "P", "P", "P", "P", "P", "P", "P", "P", "P"]], [["P", "P", "P", "P", "P", "P", "P", "P", "P", "P"], ["P", "P", "P", "P", "P", "P", "P", "P", "P", "P"], ["P", "P", "P", "P", "P", "P", "P", "P", "P", "P"], ["P", "P", "P", "P", "P", "P", "P", "P", "P", "P"]], [["P", "P", "P", "P", "P", "P", "P", "P", "P", "P"], ["P", "P", "P", "P", "P", "P", "P", "P", "P", "P"], ["P", "P", "P", "P", "P", "P", "P", "P", "P", "P"], ["P", "P", "P", "P", "P", "P", "P", "P", "P", "P"]], [["P", "P", "P", "P", "P", "P", "P", "P", "P", "P"], ["P", "P", "P", "P", "P", "P", "P", "P", "P", "P"], ["P", "P", "P", "P", "P", "P", "P", "P", "P", "P"], ["P", "P", "P", "P", "P", "P", "P", "P", "P", "P"]], [["P", "P", "P", "P", "P", "P", "P", "P", "P", "P"], ["P", "P", "P", "P", "P", "P", "P", "P", "P", "P"], ["P", "P", "P", "P", "P", "P", "P", "P", "P", "P"], ["P", "P", "P", "P", "P", "P", "P", "P", "P", "P"]], [["P", "P", "P", "P", "P", "P", "P", "P", "P", "P"], ["P", "P", "P", "P", "P", "P", "P", "P", "P", "P"], ["P", "P", "P", "P", "P", "P", "P", "P", "P", "P"], ["P", "P", "P", "P", "P", "P", "P", "P", "P", "P"]], [["P", "P", "P", "P", "P", "P", "P", "P", "P", "P"], ["P", "P", "P", "P", "P", "P", "P", "P", "P", "P"], ["P", "P", "P", "P", "P", "P", "P", "P", "P", "P"], ["P", "P", "P", "P", "P", "P", "P", "P", "P", "P"]], [["P", "P", "P", "P", "P", "P", "P", "P", "P", "P"], ["P", "P", "P", "P", "P", "P", "P", "P", "P", "P"], ["P", "P", "P", "P", "P", "P", "P", "P", "P", "P"], ["P", "P", "P", "P", "P", "P", "P", "P", "P", "P"]], [["P", "P", "P", "P", "P", "P", "P", "P", "P", "P"], ["P", "P", "P", "P", "P", "P", "P", "P", "P", "P"], ["P", "P", "P", "P", "P", "P", "P", "P", "P", "P"], ["P", "P", "P", "P", "P", "P", "P", "P", "P", "P"]], [["P", "P", "P", "P", "P", "P", "P", "P", "P", "P"], ["P", "P", "P", "P", "P", "P", "P", "P", "P", "P"], ["P", "P", "P", "P", "P", "P", "P", "P", "P", "P"], ["P", "P", "P", "P", "P", "P", "P", "P", "P", "P"]], [["P", "P", "P", "P", "P", "P", "P", "P", "P", "P"], ["P", "P", "P", "P", "P", "P", "P", "P", "P", "P"], ["P", "P", "P", "P", "P", "P", "P", "P", "P", "P"], ["P", "P", "P", "P", "P", "P", "P", "P", "P", "P"]], [["P", "P", "P", "P", "P", "P", "P", "P", "P", "P"], ["P", "P", "P", "P", "P", "P", "P", "P", "P", "P"], ["P", "P", "P", "P", "P", "P", "P", "P", "P", "P"], ["P", "P", "P", "P", "P", "P", "P", "P", "P", "P"]]]} ("clRespTime"), "RT Range"=w13, "RT_PFI"=w10, "RT Uncert"=w9) -> (→"clRespTime":T3)
